vi "_PC_Daemon_Pref objIntegration.vi"(8 "error in (no error)":errorcluster, 11 "tabObjRefnum":refnum<vi>[][](array[refnum])) -> (0 "error out":errorcluster, 1 "DI":refnum<vi>[](array[refnum]), 2 "DO":refnum<vi>[](array[refnum]), 3 "AO":refnum<vi>[](array[refnum]))   [LabVIEW 2018]
uses:
  <vilib>/regexp/Match Regular Expression.xnode
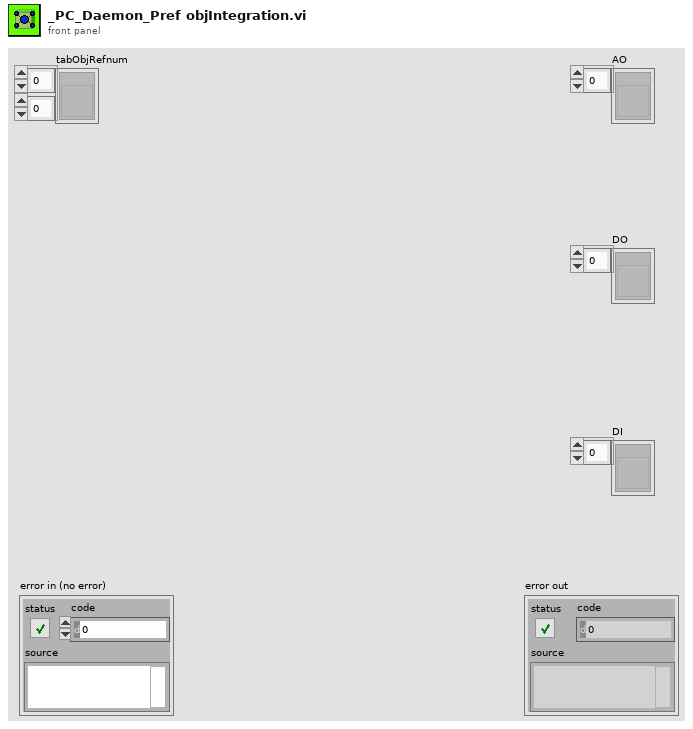
[diagram p1: front panel]
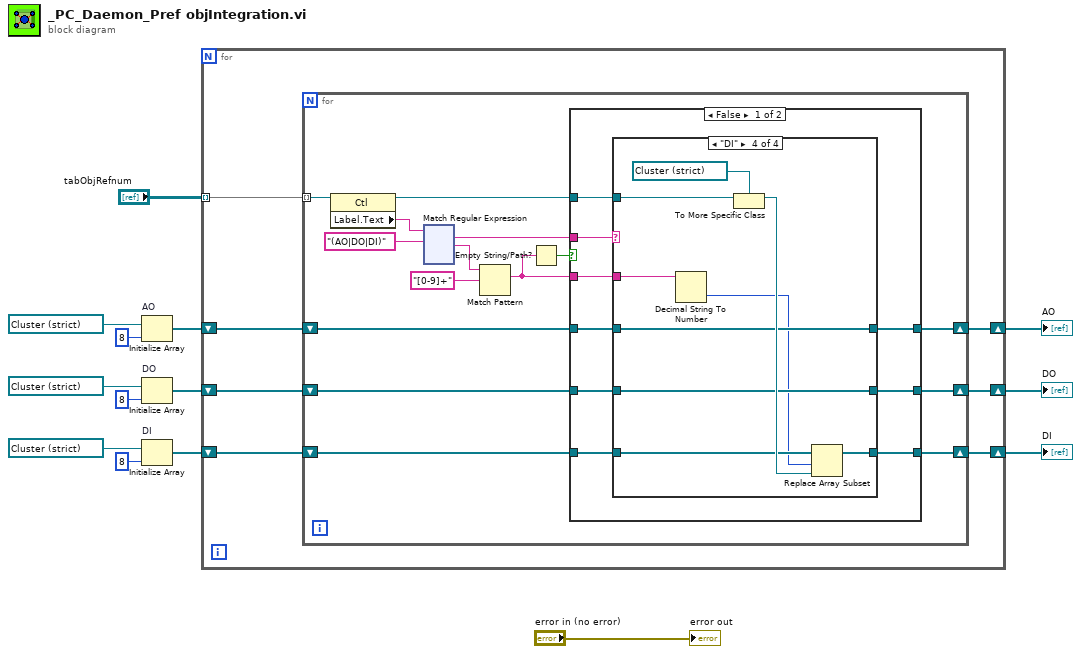
[diagram p0: block diagram]
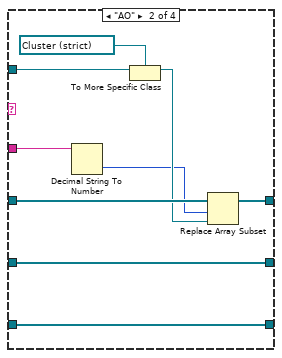
[diagram p3: hidden frame]
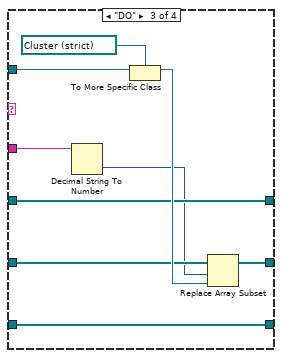
[diagram p4: hidden frame]
diagram:
  n1 = Initialize Array "AO"(refnum<vi> refnum ("AO 7"), 8 ("dimension size")) -> (w7:refnum<vi>[])
  n2 = Initialize Array "DO"(refnum<vi> refnum ("DO 7"), 8 ("dimension size")) -> (w6:refnum<vi>[])
  n3 = Initialize Array "DI"(refnum<vi> refnum ("DI 7"), 8 ("dimension size")) -> (w5:refnum<vi>[])
  n4 = for {
    tunnel: "tabObjRefnum" -> [w21] mode=indexing
    shift-right: [w16] -> w4
    shift-left: w7 -> [w20]
    shift-right: [w17] -> w3
    shift-left: w6 -> [w19]
    shift-right: [w15] -> w2
    shift-left: w5 -> [w18]
    n5 = for {
      tunnel: w21 -> [w36] mode=indexing
      shift-right: [w30] -> w16
      shift-left: w20 -> [w29]
      shift-right: [w28] -> w17
      shift-left: w19 -> [w27]
      shift-right: [w26] -> w15
      shift-left: w18 -> [w25]
      n6 = property class="Ctl"(reference=w36) -> (reference out=w22:refnum<vi>, "Label.Text"=w32:string)  [unwired: 1 in, 1 out]
      n7 = xnode "Match Regular Expression"("input string"=w32, "regular expression"="(AO|DO|DI)") -> ("whole match"=w24:string, "after match"=w34:string)  [unwired: 4 in, 3 out]
      n8 = Match Pattern(string=w34, regular expression="[0-9]+") -> (match substring=w23:string)  [unwired: 1 in, 3 out]
      n9 = Empty String/Path?(string/path=w23) -> (empty?=w31:bool)
      n10 = case shown="False" w31 {
        tunnel: [w41 w78] -> w30
        tunnel: w29 -> [w43 w78]
        tunnel: [w39 w77] -> w28
        tunnel: w27 -> [w40 w77]
        tunnel: [w37 w76] -> w26
        tunnel: w25 -> [w38 w76]
        tunnel: w24 -> [w45 _]
        tunnel: w23 -> [w44 _]
        tunnel: w22 -> [w42 _]
        frame False {
          n11 = case shown="\"DI\"" w45 {
            tunnel: w44 -> [_ w57 w66 w75]
            tunnel: w43 -> [w48 w56 w60 w68]
            tunnel: w42 -> [_ w55 w65 w74]
            tunnel: [w48 w52 w60 w68] -> w41
            tunnel: w40 -> [w47 w51 w63 w69]
            tunnel: [w47 w51 w62 w69] -> w39
            tunnel: w38 -> [w46 w50 w59 w72]
            tunnel: [w46 w50 w59 w71] -> w37
            frame Default {
            }
            frame "AO" {
              n12 = Decimal String To Number(string=w57) -> (number=w49:i32)  [unwired: 2 in, 1 out]
              n13 = To More Specific Class(target class=refnum<vi> refnum ("AO 7"), reference=w55) -> (specific class reference=w53:refnum<vi>)  [unwired: 1 in, 1 out]
              n14 = Replace Array Subset(array=w56, new element=w53, index=w49) -> (w52:refnum<vi>[])
            }
            frame "DO" {
              n15 = Decimal String To Number(string=w66) -> (number=w58:i32)  [unwired: 2 in, 1 out]
              n16 = To More Specific Class(target class=refnum<vi> refnum ("DO 7"), reference=w65) -> (specific class reference=w64:refnum<vi>)  [unwired: 1 in, 1 out]
              n17 = Replace Array Subset(array=w63, new element=w64, index=w58) -> (w62:refnum<vi>[])
            }
            frame "DI" {
              n18 = Decimal String To Number(string=w75) -> (number=w67:i32)  [unwired: 2 in, 1 out]
              n19 = To More Specific Class(target class=refnum<vi> refnum ("DI 7"), reference=w74) -> (specific class reference=w73:refnum<vi>)  [unwired: 1 in, 1 out]
              n20 = Replace Array Subset(array=w72, new element=w73, index=w67) -> (w71:refnum<vi>[])
            }
          }
        }
        frame True {
        }
      }
    }
  }
  "AO" <- w4
  "DO" <- w3
  "DI" <- w2
  "error out" <- "error in (no error)"
